vi "rszvl_core_global.vi"() -> ()   [LabVIEW 2014] (continued)
"Write Callback"="", "Range Callback"="", "Check Callback"="", "Rngtable Callback"="", "Coerce Callback"="", "User Callback"="", "Supported Models"="", "Instrument Options"="", "Repeated Capabilities"="", "Restricted Repeated Capabilities"="", "Help"="This attribute inverts the Q component of the signal.\n\nAvailable Repeated Capabilities:\nNone\n\nRemote-control command(s):\n[SENSe:]CDPower:QINVert ON | OFF", "Flags"={"OPC Wait"=FALSE, "Dont check status"=FALSE, "*WAI"=FALSE}, "Check Status Callback"=""}, {"Level"=3, "Descriptive Name"="3GPP BS Measurement WCDP Settings Power Reference", "Class Only"=FALSE, "Data Type"=0, "Access"=2, "Identifier"="RSZVL_ATTR_3GBS_WCDP_POW_REF", "Range Table"="rszvl_rng3GBSPowRef", "Command"="CDP:PREF", "Read Callback"="", "Write Callback"="", "Range Callback"="", "Check Callback"="", "Rngtable Callback"="", "Coerce Callback"="", "User Callback"="", "Supported Models"="", "Instrument Options"="", "Repeated Capabilities"="", "Restricted Repeated Capabilities"="", "Help"="This attribute switches between the use of total power or CPICH power as the reference for the\nrelative CDP measurement values.\n\nAvailable Repeated Capabilities:\nNone\n\nRemote-control command(s):\n[SENSe:]CDPower:PREFerence TOTal | CPICh", "Flags"={"OPC Wait"=FALSE, "Dont check status"=FALSE, "*WAI"=FALSE}, "Check Status Callback"=""}, {"Level"=3, "Descriptive Name"="3GPP BS Measurement WCDP Settings Inactive Channel Treshold", "Class Only"=FALSE, "Data Type"=1, "Access"=2, "Identifier"="RSZVL_ATTR_3GBS_WCDP_INACT_CHAN_THR", "Range Table"="rszvl_rng3GPPThr", "Command"="CDP:ICTR", "Read Callback"="", "Write Callback"="", "Range Callback"="", "Check Callback"="", "Rngtable Callback"="", "Coerce Callback"="", "User Callback"="", "Supported Models"="", "Instrument Options"="", "Repeated Capabilities"="", "Restricted Repeated Capabilities"="", "Help"="This attribute sets the threshold value from which a channel is treated as active. The level entered\nrefers to the total signal power.\n\nAvailable Repeated Capabilities:\nNone\n\nRemote-control command(s):\n[SENSe:]CDPower:ICTReshold", "Flags"={"OPC Wait"=FALSE, "Dont check status"=FALSE, "*WAI"=FALSE}, "Check Status Callback"=""}, {"Level"=2, "Descriptive Name"="Settings", "Class Only"=TRUE, "Data Type"=0, "Access"=0, "Identifier"="", "Range Table"="", "Command"="", "Read Callback"="", "Write Callback"="", "Range Callback"="", "Check Callback"="", "Rngtable Callback"="", "Coerce Callback"="", "User Callback"="", "Supported Models"="", "Instrument Options"="", "Repeated Capabilities"="", "Restricted Repeated Capabilities"="", "Help"="Attributes that configure the common settings.\n\n(1) 3GPP BS Settings Antenna:\nThis attribute activates or deactivates the antenna diversity mode and selects the antenna to be used.\n\nOFF The antenna diversity mode is switched off.\n1 | 2 The antenna diversity mode is switched on, and the signal from antenna 1 or antenna 2 is\nused for CDP analysis.\n\n(2) 3GPP BS Marker To Channel:\nThis attribute sets the marker to channel 0.\nThis attribute is an <Event> and, therefore, has neither an *RST value nor a query. Only the\nnumeric suffix 1 is permissible in MARKer.\nThe numeric suffix in CALCulate that is required or permissible depends on the selected display\nmode for which the marker is to be valid and has to coincide with:\nCALCulate<1> for CDP absolute and relative\nCALCulate2 for composite EVM, peak code domain error, power versus slot, bit stream,\nsymbol constellation and EVM\n\n(3) 3GPP BS Delta Marker To Channel:\nThis attribute changes the delta marker position to certain channels in code domain power measurement mode.\n\n\n(4) 3GPP BS Settings Scrambling Code:\nThis attribute defines the scrambling code in hexadecimal format.\n\n(5) 3GPP BS Timing Offset:\nThis attribute specifies whether the timing offset and pilot length are measured or if the values are\ntaken from the predefined table.\n\n(6) 3GPP BS Y axis Scaling:\nThis attribute defines the scaling of the y–axis in the currently selected unit.\n\n(7) 3GPP BS Auto Level and Code:\nThis attribute starts the following sequence:\n- Adjusts the reference level.\n- Searches automatically the scrambling code that leads to the highest signal power and stores it\nas new scrambling code.\n- Changes into the Result Summary result display.\n\n(8) 3GPP BS Scrambling Code Search:\nThis attribute searches automatically the scrambling code that leads to the highest signal power and stores it as new scrambling code for further measurements.", "Flags"={"OPC Wait"=FALSE, "Dont check status"=FALSE, "*WAI"=FALSE}, "Check Status Callback"=""}, {"Level"=3, "Descriptive Name"="3GPP BS Settings Antenna", "Class Only"=FALSE, "Data Type"=0, "Access"=2, "Identifier"="RSZVL_ATTR_3GBS_ANTENNA", "Range Table"="rszvl_rng3GBSAntenna", "Command"="CDP:ANT", "Read Callback"="", "Write Callback"="", "Range Callback"="", "Check Callback"="", "Rngtable Callback"="", "Coerce Callback"="", "User Callback"="", "Supported Models"="", "Instrument Options"="", "Repeated Capabilities"="", "Restricted Repeated Capabilities"="", "Help"="This attribute activates or deactivates the antenna diversity mode and selects the antenna to be used.\n\nOFF The antenna diversity mode is switched off.\n1 | 2 The antenna diversity mode is switched on, and the signal from antenna 1 or antenna 2 is\nused for CDP analysis.\n\nAvailable Repeated Capabilities:\nNone\n\nRemote-control command(s):\n[SENSe<1|2>:]CDPower:ANTenna OFF | 1 | 2", "Flags"={"OPC Wait"=FALSE, "Dont check status"=FALSE, "*WAI"=FALSE}, "Check Status Callback"=""}, {"Level"=3, "Descriptive Name"="3GPP BS Marker To Channel", "Class Only"=FALSE, "Data Type"=4, "Access"=1, "Identifier"="RSZVL_ATTR_3GBS_MARKER_TO_CHANNEL", "Range Table"="", "Command"="CALC:MARK:FUNC:{3GPPChannel}", "Read Callback"="", "Write Callback"="", "Range Callback"="", "Check Callback"="", "Rngtable Callback"="", "Coerce Callback"="", "User Callback"="", "Supported Models"="", "Instrument Options"="", "Repeated Capabilities"="", "Restricted Repeated Capabilities"="", "Help"="This attribute sets the marker to channel 0.\nThis attribute is an <Event> and, therefore, has neither an *RST value nor a query. Only the\nnumeric suffix 1 is permissible in MARKer.\nThe numeric suffix in CALCulate that is required or permissible depends on the selected display\nmode for which the marker is to be valid and has to coincide with:\nCALCulate<1> for CDP absolute and relative\nCALCulate2 for composite EVM, peak code domain error, power versus slot, bit stream,\nsymbol constellation and EVM\n\nAvailable Repeated Capabilities:\n3GPPChannel: Cpich,Pccpch\r\n\nRemote-control command(s):\nCALCulate<1|2>:MARKer<1>:FUNCtion:CPICh | PCCPch", "Flags"={"OPC Wait"=FALSE, "Dont check status"=FALSE, "*WAI"=FALSE}, "Check Status Callback"=""}, {"Level"=3, "Descriptive Name"="3GPP BS Delta Marker To Channel", "Class Only"=FALSE, "Data Type"=4, "Access"=1, "Identifier"="RSZVL_ATTR_3GBS_REFERENCE_MARKER_TO_CHANNEL", "Range Table"="", "Command"="CALC:DELT:FUNC:{3GPPChannel}", "Read Callback"="", "Write Callback"="", "Range Callback"="", "Check Callback"="", "Rngtable Callback"="", "Coerce Callback"="", "User Callback"="", "Supported Models"="", "Instrument Options"="", "Repeated Capabilities"="", "Restricted Repeated Capabilities"="", "Help"="This attribute changes the delta marker position to certain channels in code domain power measurement mode.\n\nAvailable Repeated Capabilities:\n3GPPChannel: Cpich,Pccpch\r\n\nRemote-control command(s):\nCALCulate<1|2>:DELTamarker<1..4>:FUNCtion:CPICh | PCCPch", "Flags"={"OPC Wait"=FALSE, "Dont check status"=FALSE, "*WAI"=FALSE}, "Check Status Callback"=""}, {"Level"=3, "Descriptive Name"="3GPP BS Settings Scrambling Code", "Class Only"=FALSE, "Data Type"=0, "Access"=2, "Identifier"="RSZVL_ATTR_3GBS_SCODE", "Range Table"="rszvl_rng3GUECDPScrCode", "Command"="CDP:LCOD", "Read Callback"="rszvl_hex_ReadCallback.vi", "Write Callback"="rszvl_hex_WriteCallback.vi", "Range Callback"="", "Check Callback"="", "Rngtable Callback"="", "Coerce Callback"="", "User Callback"="", "Supported Models"="", "Instrument Options"="", "Repeated Capabilities"="", "Restricted Repeated Capabilities"="", "Help"="This attribute defines the scrambling code in hexadecimal format.\n\nAvailable Repeated Capabilities:\nNone\n\nRemote-control command(s):\n[SENSe:]CDPower:LCODe[:VALue]", "Flags"={"OPC Wait"=FALSE, "Dont check status"=FALSE, "*WAI"=FALSE}, "Check Status Callback"=""}, {"Level"=3, "Descriptive Name"="3GPP BS Y axis Scaling", "Class Only"=FALSE, "Data Type"=1, "Access"=2, "Identifier"="RSZVL_ATTR_3GPP_PDIV", "Range Table"="", "Command"="DISP:TRAC:Y:PDIV", "Read Callback"="", "Write Callback"="", "Range Callback"="", "Check Callback"="", "Rngtable Callback"="", "Coerce Callback"="", "User Callback"="", "Supported Models"="", "Instrument Options"="", "Repeated Capabilities"="", "Restricted Repeated Capabilities"="", "Help"="This attribute defines the scaling of the y–axis in the currently selected unit.\n\nAvailable Repeated Capabilities:\nNone\n\nRemote-control command(s):\nDISPlay[:WINDow<1|2>]:TRACE<1...4>:Y[:SCALe]:PDIVision", "Flags"={"OPC Wait"=FALSE, "Dont check status"=FALSE, "*WAI"=FALSE}, "Check Status Callback"=""}, {"Level"=3, "Descriptive Name"="3GPP BS Auto Level and Code", "Class Only"=FALSE, "Data Type"=4, "Access"=1, "Identifier"="RSZVL_ATTR_3GPP_ASEQ", "Range Table"="", "Command"="CDP:ASEQ", "Read Callback"="", "Write Callback"="", "Range Callback"="", "Check Callback"="", "Rngtable Callback"="", "Coerce Callback"="", "User Callback"="", "Supported Models"="", "Instrument Options"="", "Repeated Capabilities"="", "Restricted Repeated Capabilities"="", "Help"="This attribute starts the following sequence:\n- Adjusts the reference level.\n- Searches automatically the scrambling code that leads to the highest signal power and stores it\nas new scrambling code.\n- Changes into the Result Summary result display.\n\nAvailable Repeated Capabilities:\nNone\n\nRemote-control command(s):\n[SENSe<1|2>:]CDPower:ASEQuence", "Flags"={"OPC Wait"=TRUE, "Dont check status"=FALSE, "*WAI"=FALSE}, "Check Status Callback"=""}, {"Level"=3, "Descriptive Name"="3GPP BS Scrambling Code Search", "Class Only"=FALSE, "Data Type"=4, "Access"=1, "Identifier"="RSZVL_ATTR_3GPP_SCODE_SEARCH", "Range Table"="", "Command"="CDP:LCOD:SEAR", "Read Callback"="", "Write Callback"="", "Range Callback"="", "Check Callback"="", "Rngtable Callback"="", "Coerce Callback"="", "User Callback"="", "Supported Models"="", "Instrument Options"="", "Repeated Capabilities"="", "Restricted Repeated Capabilities"="", "Help"="This attribute searches automatically the scrambling code that leads to the highest signal power and stores it as new scrambling code for further measurements.\n\nAvailable Repeated Capabilities:\nNone\n\nRemote-control command(s):\n[SENSe<1|2>:]CDPower:LCODe:SEARch[:IMMediate]", "Flags"={"OPC Wait"=TRUE, "Dont check status"=FALSE, "*WAI"=FALSE}, "Check Status Callback"=""}, {"Level"=3, "Descriptive Name"="3GPP BS Spectrum Emission Mask Select Limit Line", "Class Only"=FALSE, "Data Type"=0, "Access"=2, "Identifier"="RSZVL_ATTR_3GPP_ESP_LIMIT_LINE_SELECT", "Range Table"="rszvl_rng3GPPESPMode", "Command"="CALC:LIM:ESP:MODE", "Read Callback"="", "Write Callback"="", "Range Callback"="", "Check Callback"="", "Rngtable Callback"="", "Coerce Callback"="", "User Callback"="", "Supported Models"="", "Instrument Options"="", "Repeated Capabilities"="", "Restricted Repeated Capabilities"="", "Help"="This attribute activates or deactivates automatic selection of the limit line in the spectrum emission mask measurement.\n\nAvailable Repeated Capabilities:\nNone\n\nRemote-control command(s):\nCALCulate<1|2>:LIMit<1...8>:ESPectrum:MODE AUTO | MANual | USER", "Flags"={"OPC Wait"=FALSE, "Dont check status"=FALSE, "*WAI"=FALSE}, "Check Status Callback"=""}, {"Level"=3, "Descriptive Name"="3GPP BS Spectrum Emission Mask Predefined Limit Line", "Class Only"=FALSE, "Data Type"=0, "Access"=2, "Identifier"="RSZVL_ATTR_3GPP_ESP_PREDEFINED_LIMIT_LINE", "Range Table"="rszvl_rng3GPPESPPredefinedLimLine", "Command"="CALC:LIM:ESP:VAL", "Read Callback"="", "Write Callback"="", "Range Callback"="", "Check Callback"="", "Rngtable Callback"="", "Coerce Callback"="", "User Callback"="", "Supported Models"="", "Instrument Options"="", "Repeated Capabilities"="", "Restricted Repeated Capabilities"="", "Help"="This attribute selects one of the following predefined limit lines. As a prerequisite, the predefined limit lines must be activated using the CALCulate<1|2>:LIMit<1...8>:ESPectrum:MODE command.\n\nAvailable Repeated Capabilities:\nNone\n\nRemote-control command(s):\nCALCulate<1|2>:LIMit<1...8>:ESPectrum:VALue", "Flags"={"OPC Wait"=FALSE, "Dont check status"=FALSE, "*WAI"=FALSE}, "Check Status Callback"=""}, {"Level"=3, "Descriptive Name"="3GPP BS Spectrum Emission Mask Transition", "Class Only"=FALSE, "Data Type"=1, "Access"=2, "Identifier"="RSZVL_ATTR_3GPP_ESP_TRANSITION", "Range Table"="rszvl_rng3GPESPTransition", "Command"="CALC:LIM:ESP:TRAN", "Read Callback"="", "Write Callback"="", "Range Callback"="", "Check Callback"="", "Rngtable Callback"="", "Coerce Callback"="", "User Callback"="", "Supported Models"="", "Instrument Options"="", "Repeated Capabilities"="", "Restricted Repeated Capabilities"="", "Help"="This attribute defines the offset frequency at which the resolution bandwidth is changed.\n\nAvailable Repeated Capabilities:\nNone\n\nRemote-control command(s):\nCALCulate<1|2>:LIMit<1...8>:ESPectrum:TRANsition", "Flags"={"OPC Wait"=FALSE, "Dont check status"=FALSE, "*WAI"=FALSE}, "Check Status Callback"=""}, {"Level"=3, "Descriptive Name"="3GPP BS Spectrum Emission Mask Restore Limit Line", "Class Only"=FALSE, "Data Type"=4, "Access"=1, "Identifier"="RSZVL_ATTR_3GPP_ESP_LIMIT_LINE_RESTORE", "Range Table"="", "Command"="CALC:LIM:ESP:REST", "Read Callback"="", "Write Callback"="", "Range Callback"="", "Check Callback"="", "Rngtable Callback"="", "Coerce Callback"="", "User Callback"="", "Supported Models"="", "Instrument Options"="", "Repeated Capabilities"="", "Restricted Repeated Capabilities"="", "Help"="This attribute restores the standard limit lines for the spectrum emission mask measurement. All modifications made to the standard limit lines are lost and the factory – set values are restored.\n\nAvailable Repeated Capabilities:\nNone\n\nRemote-control command(s):\nCALCulate<1|2>:LIMit<1...8>:ESPectrum:RESTore", "Flags"={"OPC Wait"=FALSE, "Dont check status"=FALSE, "*WAI"=FALSE}, "Check Status Callback"=""}, {"Level"=2, "Descriptive Name"="Results", "Class Only"=TRUE, "Data Type"=0, "Access"=0, "Identifier"="", "Range Table"="", "Command"="", "Read Callback"="", "Write Callback"="", "Range Callback"="", "Check Callback"="", "Rngtable Callback"="", "Coerce Callback"="", "User Callback"="", "Supported Models"="", "Instrument Options"="", "Repeated Capabilities"="", "Restricted Repeated Capabilities"="", "Help"="Attributes that returns the measurement results.\n\n(1) 3GPP BS Results Spreading Factor:\nThis attribute defines the spreading factor. The spreading factor is only significant for display mode PEAK CODE DOMAIN ERROR.\n\n(2) 3GPP BS Results Select Channel:\nThis attribute sets the code number. The code number refers to code class 9 (spreading factor 512).\n\n(3) 3GPP BS Results Select CPICH Slot:\nThis attribute sets the slot number of the common pilot channels (CPICH).\n\n(4) 3GPP BS Result Type:\nThis attribute selects the measured data to be displayed.\n\n(5) 3GPP BS Result Summary View:\nThis attribute sets the view of the Code Domain Result Summary.", "Flags"={"OPC Wait"=FALSE, "Dont check status"=FALSE, "*WAI"=FALSE}, "Check Status Callback"=""}, {"Level"=3, "Descriptive Name"="3GPP BS Results Select Channel", "Class Only"=FALSE, "Data Type"=0, "Access"=2, "Identifier"="RSZVL_ATTR_3GBS_RESULTS_SELECT_CHAN", "Range Table"="rszvl_rng3GBSChannel", "Command"="CDP:CODE", "Read Callback"="", "Write Callback"="", "Range Callback"="", "Check Callback"="", "Rngtable Callback"="", "Coerce Callback"="", "User Callback"="", "Supported Models"="", "Instrument Options"="", "Repeated Capabilities"="", "Restricted Repeated Capabilities"="", "Help"="This attribute sets the code number. The code number refers to code class 9 (spreading factor 512).\n\nAvailable Repeated Capabilities:\nNone\n\nRemote-control command(s):\n[SENSe:]CDPower:CODE", "Flags"={"OPC Wait"=FALSE, "Dont check status"=FALSE, "*WAI"=FALSE}, "Check Status Callback"=""}, {"Level"=3, "Descriptive Name"="3GPP BS Results Select CPICH Slot", "Class Only"=FALSE, "Data Type"=0, "Access"=2, "Identifier"="RSZVL_ATTR_3GBS_RESULTS_SELECT_CPICH_SLOT", "Range Table"="rszvl_rng3GPPSlotNum", "Command"="CDP:SLOT", "Read Callback"="", "Write Callback"="", "Range Callback"="", "Check Callback"="", "Rngtable Callback"="", "Coerce Callback"="", "User Callback"="", "Supported Models"="", "Instrument Options"="", "Repeated Capabilities"="", "Restricted Repeated Capabilities"="", "Help"="This attribute sets the slot number of the common pilot channels (CPICH).\n\nAvailable Repeated Capabilities:\nNone\n\nRemote-control command(s):\n[SENSe:]CDPower:SLOT", "Flags"={"OPC Wait"=FALSE, "Dont check status"=FALSE, "*WAI"=FALSE}, "Check Status Callback"=""}, {"Level"=3, "Descriptive Name"="3GPP BS Result Type", "Class Only"=FALSE, "Data Type"=0, "Access"=2, "Identifier"="RSZVL_ATTR_3GBS_RESULT", "Range Table"="rszvl_rng3GBSFeed", "Command"="CALC:FEED", "Read Callback"="", "Write Callback"="", "Range Callback"="", "Check Callback"="", "Rngtable Callback"="", "Coerce Callback"="", "User Callback"="", "Supported Models"="", "Instrument Options"="", "Repeated Capabilities"="", "Restricted Repeated Capabilities"="", "Help"="This attribute selects the measured data to be displayed.\n\nAvailable Repeated Capabilities:\nNone\n\nRemote-control command(s):\nCALCulate<1|2>:FEED", "Flags"={"OPC Wait"=FALSE, "Dont check status"=FALSE, "*WAI"=FALSE}, "Check Status Callback"=""}, {"Level"=3, "Descriptive Name"="3GPP BS Result Summary View", "Class Only"=FALSE, "Data Type"=0, "Access"=2, "Identifier"="RSZVL_ATTR_3GBS_RESULT_SUM_VIEW", "Range Table"="rszvl_rng3GPPResultSumView", "Command"="CDP:RSUM", "Read Callback"="", "Write Callback"="", "Range Callback"="", "Check Callback"="", "Rngtable Callback"="", "Coerce Callback"="", "User Callback"="", "Supported Models"="", "Instrument Options"="", "Repeated Capabilities"="", "Restricted Repeated Capabilities"="", "Help"="This attribute sets the view of the Code Domain Result Summary.\n\nAvailable Repeated Capabilities:\nNone\n\nRemote-control command(s):\n[SENSe<1|2>:]CDPower:RSUMmary NORMal| EXTended", "Flags"={"OPC Wait"=FALSE, "Dont check status"=FALSE, "*WAI"=FALSE}, "Check Status Callback"=""}, {"Level"=1, "Descriptive Name"="K91 - WLAN", "Class Only"=TRUE, "Data Type"=0, "Access"=0, "Identifier"="", "Range Table"="", "Command"="", "Read Callback"="", "Write Callback"="", "Range Callback"="", "Check Callback"="", "Rngtable Callback"="", "Coerce Callback"="", "User Callback"="", "Supported Models"="", "Instrument Options"="", "Repeated Capabilities"="", "Restricted Repeated Capabilities"="", "Help"="This class implements attributes of option K91 - WLAN 802.11A, B, G & J TX\n\n(1) Settings (Class):\nAttributes that configure the measurement settings.\n\n(2) Display (Class):\nAttributes that configure the display.\n\n(3) Limit Settings (Class):\nAttributes that configure the limit settings.\n\n(4) Limit Results (Class):\nAttributes that return the limit results.\n\n(5) Marker Settings (Class):\nAttributes that configure the marker settings.\n\n(6) Results (Class):\nAttributes that returns measurement values.\n\n(7) Trigger Settings (Class):\nAttributes that configure the trigger.\n\n(8) Demodulation Settings (Class):\nAttributes that configure the demodulation.", "Flags"={"OPC Wait"=FALSE, "Dont check status"=FALSE, "*WAI"=FALSE}, "Check Status Callback"=""}, {"Level"=2, "Descriptive Name"="Settings", "Class Only"=TRUE, "Data Type"=0, "Access"=0, "Identifier"="", "Range Table"="", "Command"="", "Read Callback"="", "Write Callback"="", "Range Callback"="", "Check Callback"="", "Rngtable Callback"="", "Coerce Callback"="", "User Callback"="", "Supported Models"="", "Instrument Options"="", "Repeated Capabilities"="", "Restricted Repeated Capabilities"="", "Help"="Attributes that configure the measurement settings.\n\n(1) WLAN Standard:\nThis attribute specifies which Wireless LAN standard the option is configured to measure. \n\nFSQ-K90 supports \n0 - IEEE 802.11a\n\nFSQ-K91 supports \n0 - IEEE 802.11a\n1 - IEEE 802.11b\n2 - IEEE 802.11j (10 MHz)\n3 - IEEE 802.11j (20 MHz)\n4 - IEEE 802.11g\n5 - 802.11 OFDM Turbo Mode\n\n\n(2) WLAN PVT Reference Power:\nThis attribute configures R&S FS-K91 to use either mean or maximum burst power as the reference power for the 802.11b PVT measurement.\n\nNote:\n(1) This attribute is valid only when the selected standard is IEEE 802.11b.\n\n(3) WLAN PVT Results Interpreting:\nThis attribute configures how R&S FSQ-K91 will interpret the power versus time measurement\nresults.\nThe supplied string can be one of the following:\n\nIEEE 802.11b\n‘RISE - configures the measurement to be rising edge only.\n‘FALL - configures the measurement to be falling edge only.\n‘EDGE’ - configures the measurement to be rising and falling edge\n\nOthers\n‘EDGE’ - configures the measurement to be rising and falling edge.\n‘FULL’ - configures the measurement to be full burst.\n\nUse rszvl_rngWlanPvtSel and rszvl_rngWlanPvtSel_b table.\n\n(4) WLAN PVT Measurement:\nThis attribute configures the R&S FSQ-K91 measurement type to be Power Versus Time. After this command has been executed, the specified measurement will only be started when the user issues the INITiate command.\n\n(5) WLAN Spectrum Flatness:\nThis attribute configures the R&S FSQ-K91 measurement type to be Spectrum flatness. After this command has been executed, the specified measurement will only be started when the user issues the INITiate command\n\n(6) WLAN Burst Type:\nThis attribute specifies the type of burst to be analyzed. Only bursts of the specified type take part in measurement analysis.\n\n(7) WLAN PVT Sample Averaging:\nThis attribute configures the R&S FS-K91\nmeasurement type to set the burst power averaging length to the desired value. \n\nNote: \n(1) This attribute is valid only when the selected standard is IEEE 802.11b.\n\n(8) WLAN Signal Level IQ:\nThis attribute is used to specify the mean power level of the source signal as supplied to the Analyzer IQ inputs. This value will be overwritten if Auto Level is turned on.\n\n(9) WLAN Signal Level RF:\nThis attribute specifies the mean power level of the source signal as supplied to the analyzer RF input. This value will be overwritten if Auto Level is turned on.\n\n(10) WLAN Auto Level:\nThis attribute switch on or off automatic power level detection. When switched on, power level detection is performed at the start of each measurement sweep.\n\n(11) WLAN Auto Level Once:\nThis attribute performs the auto level routine immediately one time regardless of the current state of the Auto Level State\n\n(12) WLAN Configure Channel:\nThis attribute is used to specify the input channel for which measurements are to be performed. This command will automatically cause the internal measurement frequency to be recalculated.\n\n(13) WLAN EVM Versus Carrier Measurement:\nThis attribute configures the R&S FSQ-K91 measurement type to be EVM Versus Carrier. After this command has been executed, the specified measurement will only be started when the user issues the INITiate command.\n\n(14) WLAN EVM Versus Symbol Measurement:\nThis attribute configures the FSQ-K91 measurement type to be EVM Versus Symbol. After this command has been executed, the specified measurement will only be started when the user issues the INITiate command\n\n(15) WLAN Spectrum MASK:\nThis attribute configures the R&S FSQ-K91 measurement type to be Spectrum mask. After this command has been executed, the specified measurement will only be started when the user issues the INITiate command\n\n(16) WLAN Spectrum MASK Select:\nThis attribute configures how R&S FS-K91 will interpret the Spectrum MASK measurement results.\nThis is either performed using the IEEE or ETSI standard. \n\nNote:\n(1) This attribute is only available for IEEE\n802.11a.\n\n(17) WLAN Spectrum FFT:\nThis attribute configures the R&S FSQ-K91 measurement type to be FFT (Fast Fourier Transform). After this command has been executed, the specified measurement will only be started when the user issues the INITiate command\n\n(18) WLAN Spectrum ACPR:\nThis attribute configures the R&S FSQ-K91/K92 measurement type to be ACPR (adjacent channel power ratio). After this command has been executed, the specified measurement will only be started when the user issues the INITiate command\n\n(19) WLAN Constelation Versus Symbol:\nThis attribute configures the R&S FSQ-K91 measurement type to be Constellation versus Symbol. After this command has been executed, the specified measurement will only be started when the user issues the INITiate command\n\n(20) WLAN Overall Burst Count:\nWhen this attribute is set to on, the burst count parameter will be used by the measurement,\notherwise the burst count parameter will be ignored.\n\n(21) WLAN Constelation Versus Carrier:\nThis attribute configures the R&S FSQ-K91 measurement type to be Constellation versus Carrier. After this command has been executed, the specified\nmeasurement will only be started when the user issues the INITiate command.\n\n(22) WLAN Constellation Carrier Select:\nThis attribute is only available when Constellation versus Symbol measurement is selected. When the Constellation versus Symbol measurement is initiated, it will calculate the results of the selected carrier.\n\nNote:\n(1) This attribute is not available for IEEE 802.11b standard.\n\n(23) WLAN Constellation Carrier Select Num:\nThis attribute is only available when Constellation versus Symbol measurement is selected. When the Constellation versus Symbol measurement is initiated, it will calculate the results of the selected carrier.\n\nNote:¨\n(1) This attribute is not available for IEEE 802.11b standard.\n\n(2) Values -26 to 26 exclude 0 are available\n\n(24) WLAN Statistics CCDF:\nThis attribute configures the R&S FSQ-K91 measurement type to be CCDF (conditional cumulative distribution functions.). After this command has been executed, the specified measurement will only be started when the user issues the INITiate command\n\n(25) WLAN Statistics Bit Stream:\nThis attribute configures the R&S FSQ-K91 measurement type to be bit stream. After this command has been executed, the specified measurement will only be started when the user issues the INITiate command\n\n(26) WLAN Statistics Signal Field:\nThis attribute configures the R&S FS-K91 measurement type to be signal field. After this command has been executed, the specified measurement will only be started when the user issues the INITiate command.\n\n(27) WLAN Start Measurement:\nThis attribute requests the R&S FSQ-K91 option to start a new measurement sequence. If a measurement sequence is already in progress, the command will be ignored.\n\n(28) WLAN Run Continuous:\nThis attribute determines whether the trigger system is continuously initiated (continuous) or\nperforms single measurements (single).\n\n(29) WLAN Mode:\nThis attribute selects active operation of the R&S FSQ-K91 option by specifying its name.\n\n(30) WLAN Number of Burst:\nThis attribute defines the number of bursts that will be analyzed by the measurement. This attribute is not valid, if the setting for the [SENSe:]BURst:COUNt:STATe parameter is off.\n\n(31) WLAN Swap IQ:\nThis attribute defines whether or not the recorded IQ pairs should be swapped (I/Q) before being processed.\n\n(32) WLAN ACP Mode:\nThis attribut sets the ACP measurement mode to either absolute or relative.\n\nNote:\n(1) This attribute is available only for IEEE 802.11j standard.\n\n(33) WLAN Preamble Unit:\nThis attribute specifies the units for Preamble error results.\n\n\n(34) WLAN EVM Unit:\nThis attribute specifies the units for EVM trace results.\n\n\n(35) WLAN Gain Imbalance Unit:\nThis attribute specifies the units for gain imbalance results.\n\n(36) WLAN Phase or Frequency vs Preamble:\nThis attribute configures the R&S FSQ-K90/K91 measurement type to be Phase or Frequency Vs Premable. After this command has been executed, the specified measurement will only be started when the user issues the INITiate command\n\n(37) WLAN IQ Sample Rate:\nThis attribute allows the sample rate for IQ measurements to be specified. \n\nValid Range: 10.0e3 Hz to 100.0e6 Hz (326.4e6 Hz with option R&S FSQ-B72)\n\n(38) WLAN IQ Filter Flatness:\nThis attribute determines whether the wideband detector filters are to be used in preference to\nthe wideband detector board, (B72 option), for a specified sample rate.\n\n(39) WLAN Automatic Power Level Sweep Time:\nThis attribute specifies the sweep time for the automatic power level detection.\n\n(40) WLAN Load IQ Data:\nThis attribute loads IQ data from the specified .iqw file.\n\n(41) WLAN Save IQ Data:\nThis attribute stores IQ data to the specified .iqw file.\n\n(42) WLAN Burst Recalculate:\nThis attribute forces the IQ measurement results to be recalculated according to the current settings\n\n(43) WLAN Preamble Select:\nThis attribute specifies whether Frequency or Phase results are displayed when the\nmeasurement type is set to Error Vs Preamble", "Flags"={"OPC Wait"=FALSE, "Dont check status"=FALSE, "*WAI"=FALSE}, "Check Status Callback"=""}, {"Level"=3, "Descriptive Name"="WLAN Standard", "Class Only"=FALSE, "Data Type"=0, "Access"=2, "Identifier"="RSZVL_ATTR_WLAN_STAN", "Range Table"="rszvl_rngWlanStandard", "Command"="CONF:STAN", "Read Callback"="", "Write Callback"="", "Range Callback"="", "Check Callback"="", "Rngtable Callback"="", "Coerce Callback"="", "User Callback"="", "Supported Models"="", "Instrument Options"="", "Repeated Capabilities"="", "Restricted Repeated Capabilities"="", "Help"="This attribute specifies which Wireless LAN standard the option is configured to measure. \n\n0 - IEEE 802.11a\n1 - IEEE 802.11b\n2 - IEEE 802.11j (10 MHz)\n3 - IEEE 802.11j (20 MHz)\n4 - IEEE 802.11g\n\nAvailable Repeated Capabilities:\nNone\n\nRemote-control command(s):\nCONFigure:STANdard", "Flags"={"OPC Wait"=FALSE, "Dont check status"=FALSE, "*WAI"=FALSE}, "Check Status Callback"=""}, {"Level"=3, "Descriptive Name"="WLAN PVT Reference Power", "Class Only"=FALSE, "Data Type"=0, "Access"=2, "Identifier"="RSZVL_ATTR_WLAN_PVT_RPOW", "Range Table"="rszvl_rngWlanPvtRPow", "Command"="CONF:BURS:PVT:RPOW", "Read Callback"="", "Write Callback"="", "Range Callback"="", "Check Callback"="", "Rngtable Callback"="", "Coerce Callback"="", "User Callback"="", "Supported Models"="", "Instrument Options"="", "Repeated Capabilities"="", "Restricted Repeated Capabilities"="", "Help"="This attribute configures R&S FS-K91 to use either mean or maximum burst power as the reference power for the 802.11b PVT measurement.\n\nNote:\n(1) This attribute is valid only when the selected standard is IEEE 802.11b.\n\nAvailable Repeated Capabilities:\nNone\n\nRemote-control command(s):\nCONFigure:BURSt:PVT:RPOWer MEAN | MAX", "Flags"={"OPC Wait"=FALSE, "Dont check status"=FALSE, "*WAI"=FALSE}, "Check Status Callback"=""}, {"Level"=3, "Descriptive Name"="WLAN PVT Results Interpreting", "Class Only"=FALSE, "Data Type"=0, "Access"=2, "Identifier"="RSZVL_ATTR_WLAN_PVT_SEL", "Range Table"="rszvl_rngWlanPvtSel", "Command"="CONF:BURS:PVT:SEL", "Read Callback"="", "Write Callback"="", "Range Callback"="", "Check Callback"="", "Rngtable Callback"="", "Coerce Callback"="", "User Callback"="", "Supported Models"="", "Instrument Options"="", "Repeated Capabilities"="", "Restricted Repeated Capabilities"="", "Help"="This attribute configures how R&S FSQ-K91 will interpret the power versus time measurement\nresults.\nThe supplied string can be one of the following:\n\nIEEE 802.11b\n‘RISE - configures the measurement to be rising edge only.\n‘FALL - configures the measurement to be falling edge only.\n‘EDGE’ - configures the measurement to be rising and falling edge\n\nOthers\n‘EDGE’ - configures the measurement to be rising and falling edge.\n‘FULL’ - configures the measurement to be full burst.\n\nUse rszvl_rngWlanPvtSel and rszvl_rngWlanPvtSel_b table.\n\nAvailable Repeated Capabilities:\nNone\n\nRemote-control command(s):\nCONFigure:BURSt:PVT:SELect EDGE | FULL | RISE | FALL", "Flags"={"OPC Wait"=FALSE, "Dont check status"=FALSE, "*WAI"=FALSE}, "Check Status Callback"=""}, {"Level"=3, "Descriptive Name"="WLAN PVT Measurement", "Class Only"=FALSE, "Data Type"=4, "Access"=1, "Identifier"="RSZVL_ATTR_WLAN_PVT", "Range Table"="", "Command"="CONF:BURS:PVT", "Read Callback"="", "Write Callback"="", "Range Callback"="", "Check Callback"="", "Rngtable Callback"="", "Coerce Callback"="", "User Callback"="", "Supported Models"="", "Instrument Options"="", "Repeated Capabilities"="", "Restricted Repeated Capabilities"="", "Help"="This attribute configures the R&S FSQ-K91 measurement type to be Power Versus Time. After this command has been executed, the specified measurement will only be started when the user issues the INITiate command.\n\nAvailable Repeated Capabilities:\nNone\n\nRemote-control command(s):\nCONFigure:BURSt:PVT[:IMMediate]", "Flags"={"OPC Wait"=TRUE, "Dont check status"=FALSE, "*WAI"=FALSE}, "Check Status Callback"=""}, {"Level"=3, "Descriptive Name"="WLAN Spectrum Flatness", "Class Only"=FALSE, "Data Type"=4, "Access"=1, "Identifier"="RSZVL_ATTR_WLAN_SPEC_FLAT", "Range Table"="", "Command"="CONF:BURS:SPEC:FLAT", "Read Callback"="", "Write Callback"="", "Range Callback"="", "Check Callback"="", "Rngtable Callback"="", "Coerce Callback"="", "User Callback"="", "Supported Models"="", "Instrument Options"="", "Repeated Capabilities"="", "Restricted Repeated Capabilities"="", "Help"="This attribute configures the R&S FSQ-K91 measurement type to be Spectrum flatness. After this command has been executed, the specified measurement will only be started when the user issues the INITiate command\n\nAvailable Repeated Capabilities:\nNone\n\nRemote-control command(s):\nCONFigure:BURSt:SPECtrum:FLATness[:IMMediate]", "Flags"={"OPC Wait"=TRUE, "Dont check status"=FALSE, "*WAI"=FALSE}, "Check Status Callback"=""}, {"Level"=3, "Descriptive Name"="WLAN Burst Type", "Class Only"=FALSE, "Data Type"=0, "Access"=2, "Identifier"="RSZVL_ATTR_WLAN_BTYP", "Range Table"="rszvl_rngWlanBurstType", "Command"="DEM:FORM:BAN:BTYP", "Read Callback"="", "Write Callback"="rszvl_burstType_WriteCallback.vi", "Range Callback"="", "Check Callback"="", "Rngtable Callback"="", "Coerce Callback"="", "User Callback"="", "Supported Models"="", "Instrument Options"="", "Repeated Capabilities"="", "Restricted Repeated Capabilities"="", "Help"="This attribute specifies the type of burst to be analyzed. Only bursts of the specified type take part in measurement analysis.\n\nAvailable Repeated Capabilities:\nNone\n\nRemote-control command(s):\n[SENSe:]DEMod:FORMat:BANalyze:BTYPe", "Flags"={"OPC Wait"=FALSE, "Dont check status"=FALSE, "*WAI"=FALSE}, "Check Status Callback"=""}, {"Level"=3, "Descriptive Name"="WLAN PVT Sample Averaging", "Class Only"=FALSE, "Data Type"=0, "Access"=2, "Identifier"="RSZVL_ATTR_WLAN_PVT_AVER", "Range Table"="rszvl_rngWlanPvtSampAver", "Command"="CONF:BURS:PVT:AVER", "Read Callback"="", "Write Callback"="", "Range Callback"="", "Check Callback"="", "Rngtable Callback"="", "Coerce Callback"="", "User Callback"="", "Supported Models"="", "Instrument Options"="", "Repeated Capabilities"="", "Restricted Repeated Capabilities"="", "Help"="This attribute configures the R&S FS-K91\nmeasurement type to set the burst power averaging length to the desired value. \n\nNote: \n(1) This attribute is valid only when the selected standard is IEEE 802.11b.\n\nAvailable Repeated Capabilities:\nNone\n\nRemote-control command(s):\nCONFigure:BURSt:PVT:AVERage", "Flags"={"OPC Wait"=FALSE, "Dont check status"=FALSE, "*WAI"=FALSE}, "Check Status Callback"=""}, {"Level"=3, "Descriptive Name"="WLAN Signal Level RF", "Class Only"=FALSE, "Data Type"=1, "Access"=2, "Identifier"="RSZVL_ATTR_WLAN_POW_EXP_RF", "Range Table"="", "Command"="CONF:POW:EXP:RF", "Read Callback"="", "Write Callback"="", "Range Callback"="", "Check Callback"="", "Rngtable Callback"="", "Coerce Callback"="", "User Callback"="", "Supported Models"="", "Instrument Options"="", "Repeated Capabilities"="", "Restricted Repeated Capabilities"="", "Help"="This attribute specifies the mean power level of the source signal as supplied to the analyzer RF input. This value will be overwritten if Auto Level is turned on.\n\nAvailable Repeated Capabilities:\nNone\n\nRemote-control command(s):\nCONFigure:POWer:EXPected:RF", "Flags"={"OPC Wait"=FALSE, "Dont check status"=FALSE, "*WAI"=FALSE}, "Check Status Callback"=""}, {"Level"=3, "Descriptive Name"="WLAN Auto Level", "Class Only"=FALSE, "Data Type"=3, "Access"=2, "Identifier"="RSZVL_ATTR_WLAN_POW_AUTO", "Range Table"="", "Command"="CONF:POW:AUTO", "Read Callback"="", "Write Callback"="", "Range Callback"="", "Check Callback"="", "Rngtable Callback"="", "Coerce Callback"="", "User Callback"="", "Supported Models"="", "Instrument Options"="", "Repeated Capabilities"="", "Restricted Repeated Capabilities"="", "Help"="This attribute switch on or off automatic power level detection. When switched on, power level detection is performed at the start of each measurement sweep.\n\nAvailable Repeated Capabilities:\nNone\n\nRemote-control command(s):\nCONFigure:POWer:AUTO ON | OFF", "Flags"={"OPC Wait"=FALSE, "Dont check status"=FALSE, "*WAI"=FALSE}, "Check Status Callback"=""}, {"Level"=3, "Descriptive Name"="WLAN Auto Level Once", "Class Only"=FALSE, "Data Type"=4, "Access"=1, "Identifier"="RSZVL_ATTR_WLAN_POW_AUTO_ONCE", "Range Table"="", "Command"="CONF:POW:AUTO ONCE", "Read Callback"="", "Write Callback"="", "Range Callback"="", "Check Callback"="", "Rngtable Callback"="", "Coerce Callback"="", "User Callback"="", "Supported Models"="", "Instrument Options"="", "Repeated Capabilities"="", "Restricted Repeated Capabilities"="", "Help"="This attribute performs the auto level routine immediately one time regardless of the current state of the Auto Level State\n\nAvailable Repeated Capabilities:\nNone\n\nRemote-control command(s):\nCONFigure:POWer:AUTO ONCE", "Flags"={"OPC Wait"=FALSE, "Dont check status"=FALSE, "*WAI"=FALSE}, "Check Status Callback"=""}, {"Level"=3, "Descriptive Name"="WLAN Configure Channel", "Class Only"=FALSE, "Data Type"=0, "Access"=2, "Identifier"="RSZVL_ATTR_WLAN_CHAN", "Range Table"="", "Command"="CONF:CHAN", "Read Callback"="", "Write Callback"="", "Range Callback"="", "Check Callback"="", "Rngtable Callback"="", "Coerce Callback"="", "User Callback"="", "Supported Models"="", "Instrument Options"="", "Repeated Capabilities"="", "Restricted Repeated Capabilities"="", "Help"="This attribute is used to specify the input channel for which measurements are to be performed. This command will automatically cause the internal measurement frequency to be recalculated.\n\nAvailable Repeated Capabilities:\nNone\n\nRemote-control command(s):\nCONFigure:CHANnel", "Flags"={"OPC Wait"=FALSE, "Dont check status"=FALSE, "*WAI"=FALSE}, "Check Status Callback"=""}, {"Level"=3, "Descriptive Name"="WLAN EVM Versus Carrier Measurement", "Class Only"=FALSE, "Data Type"=4, "Access"=1, "Identifier"="RSZVL_ATTR_WLAN_EVM_ECAR", "Range Table"="", "Command"="CONF:BURS:EVM:ECAR", "Read Callback"="", "Write Callback"="", "Range Callback"="", "Check Callback"="", "Rngtable 
